vi "串口.vi"() -> ()   [LabVIEW 2018]
uses:
  <vilib>/Instr/_visa.llb/VISA Configure Serial Port (Instr).vi
panel:
  out "波形图表":dbl(graph)
  out "*(类型 *) &3":dbl
  out "数值 2":i32
  out "数值":i32
  in  "停止":bool
  out "第一个子数组":u8[](array[numeric])
  out "布尔":bool
  out "Bytes at Port":u32
  out "错误输出":errorcluster
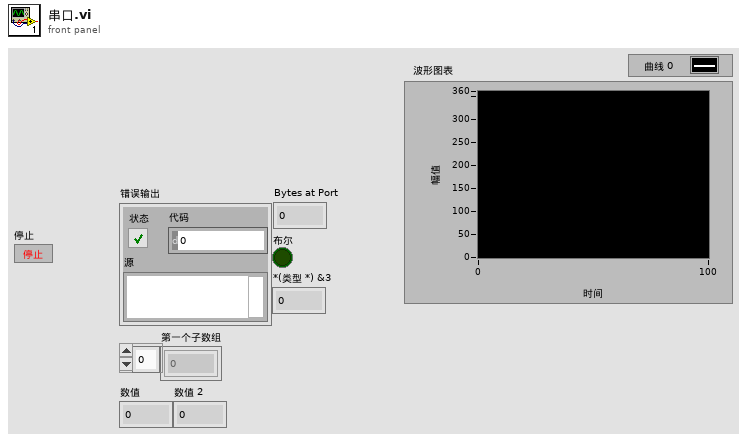
[diagram p1: front panel]
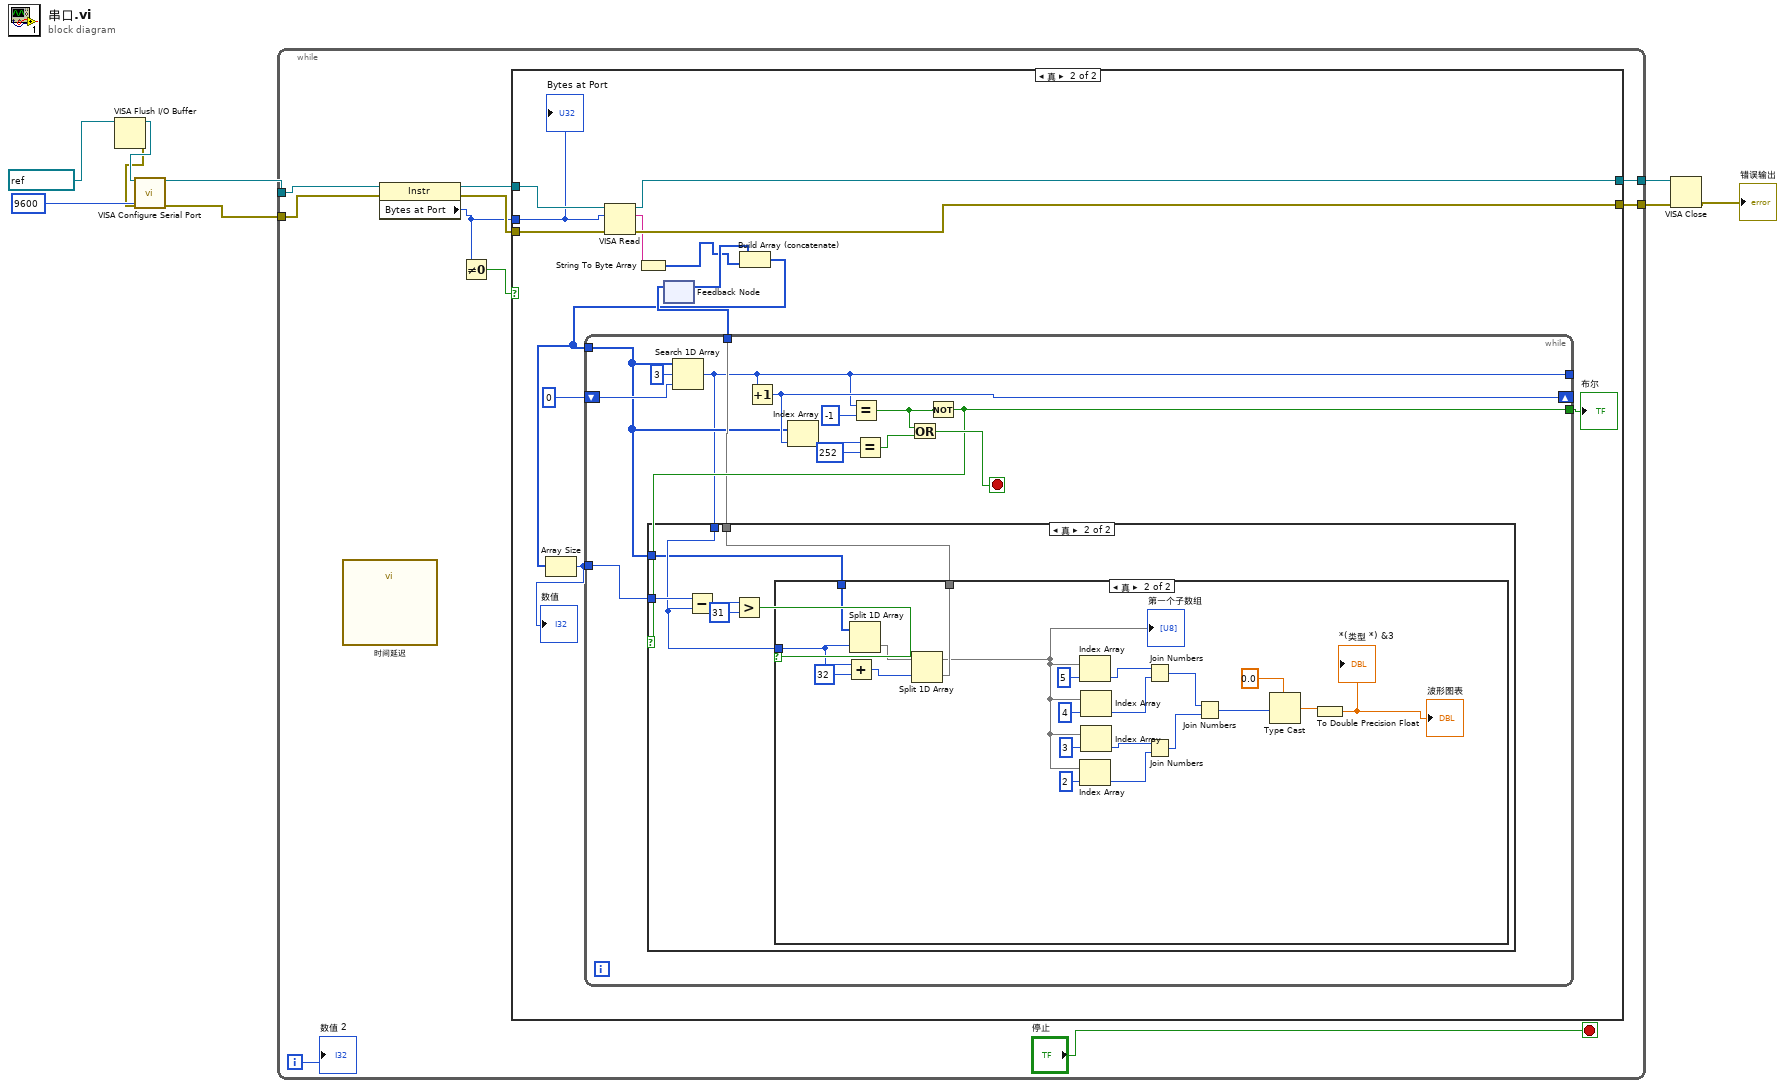
[diagram p0: block diagram]
diagram:
  n1 = VISA Flush I/O Buffer(VISA resource name=refnum<visa-resource-name> "COM6") -> (VISA resource name out=w2:refnum<visa-resource-name>, error out=w1:errorcluster)  [unwired: 2 in]
  n2 = call-poly "VISA Configure Serial Port"("VISA resource name"=w2, "baud rate (9600)"=u32 9600, "error in (no error)"=w1) -> ("VISA resource name out"=w9:refnum<visa-resource-name>, "error out"=w8:errorcluster)  [unwired: 11 in]
  n3 = while {
    tunnel: w9 -> [w19]
    tunnel: w8 -> [w18]
    tunnel: [w14] -> w5
    tunnel: [w13] -> w4
    i -> [w10]
    stop <- "停止" stop-if-true
    n4 = call "时间延迟"() -> ()  [unwired: 11 in, 1 out]
    n5 = property class="Instr"(reference=w19, error in=w18) -> (reference out=w16:refnum<visa-resource-name>, error out=w15:errorcluster, "Bytes at Port"=w12:u32)
    n6 = Not Equal To 0?(x=w12) -> (x != 0?=w17:bool)
    n7 = case shown="真" w17 {
      tunnel: w16 -> [w21 w34]
      tunnel: w15 -> [w20 w33]
      tunnel: [w21 w32] -> w14
      tunnel: [w20 w31] -> w13
      tunnel: w12 -> [_ w29]
      frame False {
      }
      frame True {
        n8 = VISA Read(VISA resource name=w34, byte count=w29, error in (no error)=w33) -> (VISA resource name out=w32:refnum<visa-resource-name>, read buffer=w30:string, error out=w31:errorcluster)  [unwired: 1 out]
        n9 = String To Byte Array(string=w30) -> (unsigned byte array=w22:u8[])
        n10 = feedback #1() -> (w24:u8[])  [unwired: 1 in]
        n11 = Build Array (concatenate)(w24, w22) -> (w23:u8[])
        n12 = Array Size(array=w23) -> (size(s)=w25:i32)
        "数值" <- w25
        n13 = while {
          shift-right: [w37] -> _
          shift-left: 0 -> [w47]
          tunnel: [w35] -> _
          tunnel: [w40] -> w27
          tunnel: [w39] -> w26
          tunnel: w25 -> [w38]
          tunnel: w23 -> [w36]
          stop <- w42 stop-if-true
          n14 = Search 1D Array(1D array=w36, element=u8 3 ("元素"), start index (0)=w47) -> (index of element=w35:i32)
          n15 = Increment(x=w35) -> (x+1=w37:i32)
          n16 = Index Array(array=w36, index=w37) -> (element=w45:u8)
          n17 = Equal?(x=w35, y=-1) -> (x = y?=w41:bool)
          n18 = Equal?(x=w45, y=u8 252) -> (x = y?=w43:bool)
          n19 = Or(x=w41, y=w43) -> (x .or. y?=w42:bool)
          n20 = Not(x=w41) -> (.not. x?=w40:bool)
          n21 = case shown="真" w40 {
            tunnel: [w49 w50] -> w39
            tunnel: w38 -> [_ w56]
            tunnel: w35 -> [_ w52]
            tunnel: w36 -> [w49 w51]
            frame False {
            }
            frame True {
              n22 = Subtract(x=w56, y=w52) -> (x-y=w55:i32)
              n23 = Greater?(x=w55, y=31) -> (0:w53:bool)
              n24 = case shown="真" w53 {
                tunnel: w52 -> [_ w76]
                tunnel: w51 -> [w57 w78]
                tunnel: [w57 w73] -> w50
                frame False {
                }
                frame True {
                  n25 = Add(x=w76, y=32) -> (x+y=w74:i32)
                  n26 = Split 1D Array(array=w78, index=w76) -> (second subarray=w77:u8[])  [unwired: 1 out]
                  n27 = Split 1D Array(array=w77, index=w74) -> (first subarray=w72:u8[], second subarray=w73:u8[])
                  "第一个子数组" <- w72
                  n28 = Index Array(array=w72, index=5 ("索引")) -> (element=w67:u8)
                  n29 = Index Array(array=w72, index=2 ("索引")) -> (element=w64:u8)
                  n30 = Index Array(array=w72, index=4 ("索引")) -> (element=w66:u8)
                  n31 = Index Array(array=w72, index=3 ("索引")) -> (element=w65:u8)
                  n32 = Join Numbers(hi=w67, lo=w66) -> ((hi.lo)=w62:u16)
                  n33 = Join Numbers(hi=w65, lo=w64) -> ((hi.lo)=w63:u16)
                  n34 = Join Numbers(hi=w62, lo=w63) -> ((hi.lo)=w60:u32)
                  n35 = Type Cast(type=sgl 0.0, x=w60) -> (*(type *) &x=w59:sgl)
                  n36 = To Double Precision Float(number=w59) -> (double precision float=→"*(类型 *) &3" →"波形图表":dbl)
                }
              }
            }
          }
        }
        "布尔" <- w27
        n37 = feedback-in #1(w26) -> ()
        "Bytes at Port" <- w29
      }
    }
    "数值 2" <- w10
  }
  n38 = VISA Close(VISA resource name=w5, error in (no error)=w4) -> (error out=→"错误输出":errorcluster)
